vi "volume.indexer.vi"() -> ()   [LabVIEW 2024]
panel:
  in  "Issue Path":path
  in  "Volume Path":path
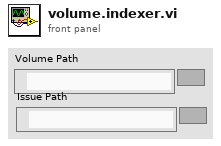
[diagram p1: front panel]
types:
  T1 = typedef "local_volume.ctl" = cluster{"id":i32, "name":string, "sortable_name":string, "aliases":string[], "description":string, "site_detail_url":string, "count_of_issues":i32, "start_year":i32, "publisher_id":i32, "issue_ids":i32[], "date_last_updated":timestamp, "volume":i32, "cv_id":string}
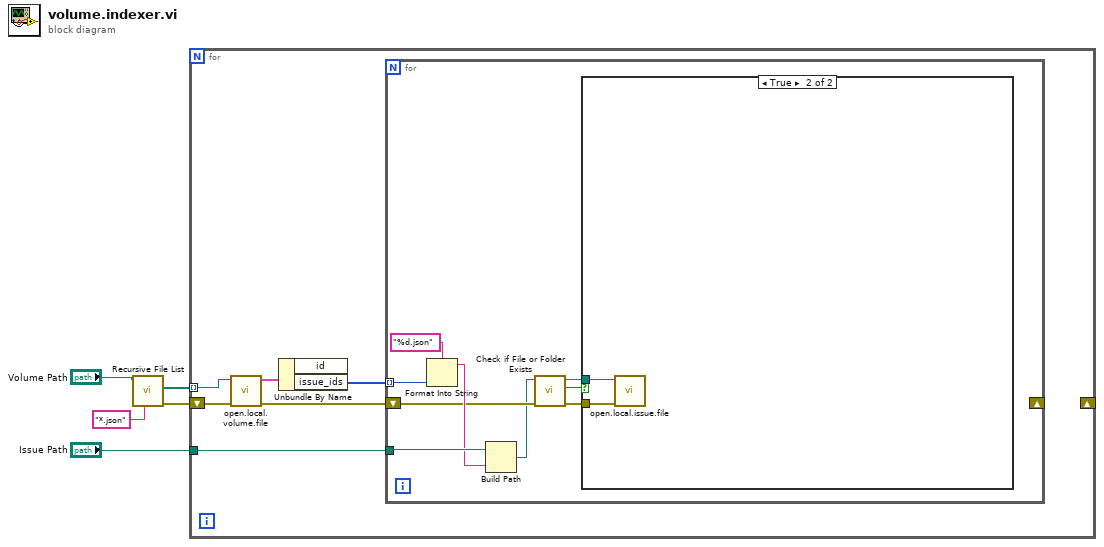
[diagram p0: block diagram]
diagram:
  n1 = call <vilib>:"Recursive File List.vi"("pattern"="*.json", "Folder Path"="Volume Path") -> ("error out"=w3:errorcluster, "All Files in Dir"=w2:path[])  [unwired: 5 in, 3 out]
  n2 = for {
    shift-right: _ -> [_]
    shift-left: w3 -> [w11]
    tunnel: w2 -> [w10] mode=indexing
    tunnel: "Issue Path" -> [w7]
    n3 = call "open.local.volume.file.vi"("error in (no error)"=w11, "volume json"=w10) -> ("error out"=w6:errorcluster, "volume"=w9:T1)  [unwired: 8 in]
    n4 = Unbundle By Name(w9) -> ("issue_ids"=w8:i32[])  [unwired: 1 out]
    n5 = for {
      tunnel: w8 -> [w19] mode=indexing
      tunnel: w7 -> [w18]
      shift-right: _ -> [_]
      shift-left: w6 -> [w16]
      n6 = Format Into String(format string="%d.json", w19) -> (resulting string=w17:string)  [unwired: 2 in, 1 out]
      n7 = Build Path(base path=w18, name or relative path=w17) -> (appended path=w15:path)
      n8 = call <vilib>:"Check if File or Folder Exists.vi"("error in (no error)"=w16, "path"=w15) -> ("error out"=w12:errorcluster, "file or folder exists?"=w14:bool, "dup path"=w13:path)  [unwired: 7 in]
      n9 = case shown="True" w14 {
        tunnel: w13 -> [_ w22]
        tunnel: w12 -> [_ w21]
        frame False {
        }
        frame True {
          n10 = call "open.local.issue.file.vi"("error in (no error)"=w21, "volume json"=w22) -> ()  [unwired: 8 in, 2 out]
        }
      }
    }
  }
